vi "Temperature Simulator.vi"() -> (3 "Temperature Value":dbl)   [LabVIEW 2018]
panel:
  in  "Upper Limit (30)":dbl=30.0
  in  "Lower Limit (20)":dbl=20.0
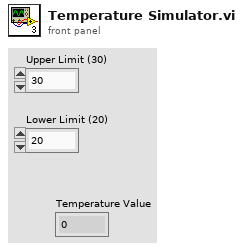
[diagram p1: front panel]
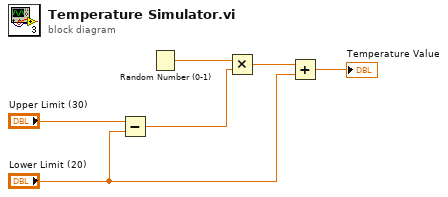
[diagram p0: block diagram]
diagram:
  n1 = Subtract(x="Upper Limit (30)", y="Lower Limit (20)") -> (x-y=w1:dbl)
  n2 = Random Number (0-1)() -> (number: 0 to 1=w2:dbl)
  n3 = Multiply(x=w2, y=w1) -> (x*y=w5:dbl)
  n4 = Add(x=w5, y="Lower Limit (20)") -> (x+y=→"Temperature Value":dbl)
